vi "data_process.vi"(0 "文件（使用对话框）":path) -> (19 "SENSOR 9":dbl[](array[numeric]), 20 "SENSOR1":dbl[](array[numeric]), 21 "SENSOR 2":dbl[](array[numeric]), 22 "SENSOR 3":dbl[](array[numeric]), 23 "SENSOR 4":dbl[](array[numeric]), 24 "SENSOR 5":dbl[](array[numeric]), 25 "SENSOR 6":dbl[](array[numeric]), 26 "SENSOR 7":dbl[](array[numeric]), 27 "SENSOR 8":dbl[](array[numeric]))   [LabVIEW 2017]
panel:
  out "PWM19":dbl[](array[numeric])
  out "PWM18":dbl[](array[numeric])
  out "PWM17":dbl[](array[numeric])
  out "PWM16":dbl[](array[numeric])
  out "PWM15":dbl[](array[numeric])
  out "PWM14":dbl[](array[numeric])
  out "PWM13":dbl[](array[numeric])
  out "PWM12":dbl[](array[numeric])
  out "PWM11":dbl[](array[numeric])
  out "PWM10":dbl[](array[numeric])
  out "PWM9":dbl[](array[numeric])
  out "PWM8":dbl[](array[numeric])
  out "PWM7":dbl[](array[numeric])
  out "PWM6":dbl[](array[numeric])
  out "PWM5":dbl[](array[numeric])
  out "PWM4":dbl[](array[numeric])
  out "PWM3":dbl[](array[numeric])
  out "匹配偏移量":i32
  out "PWM2":dbl[](array[numeric])
  out "文本":string
  out "PWM1":dbl[](array[numeric])
  # "主要功能：将9行数据分别提取出来作为一个列表"
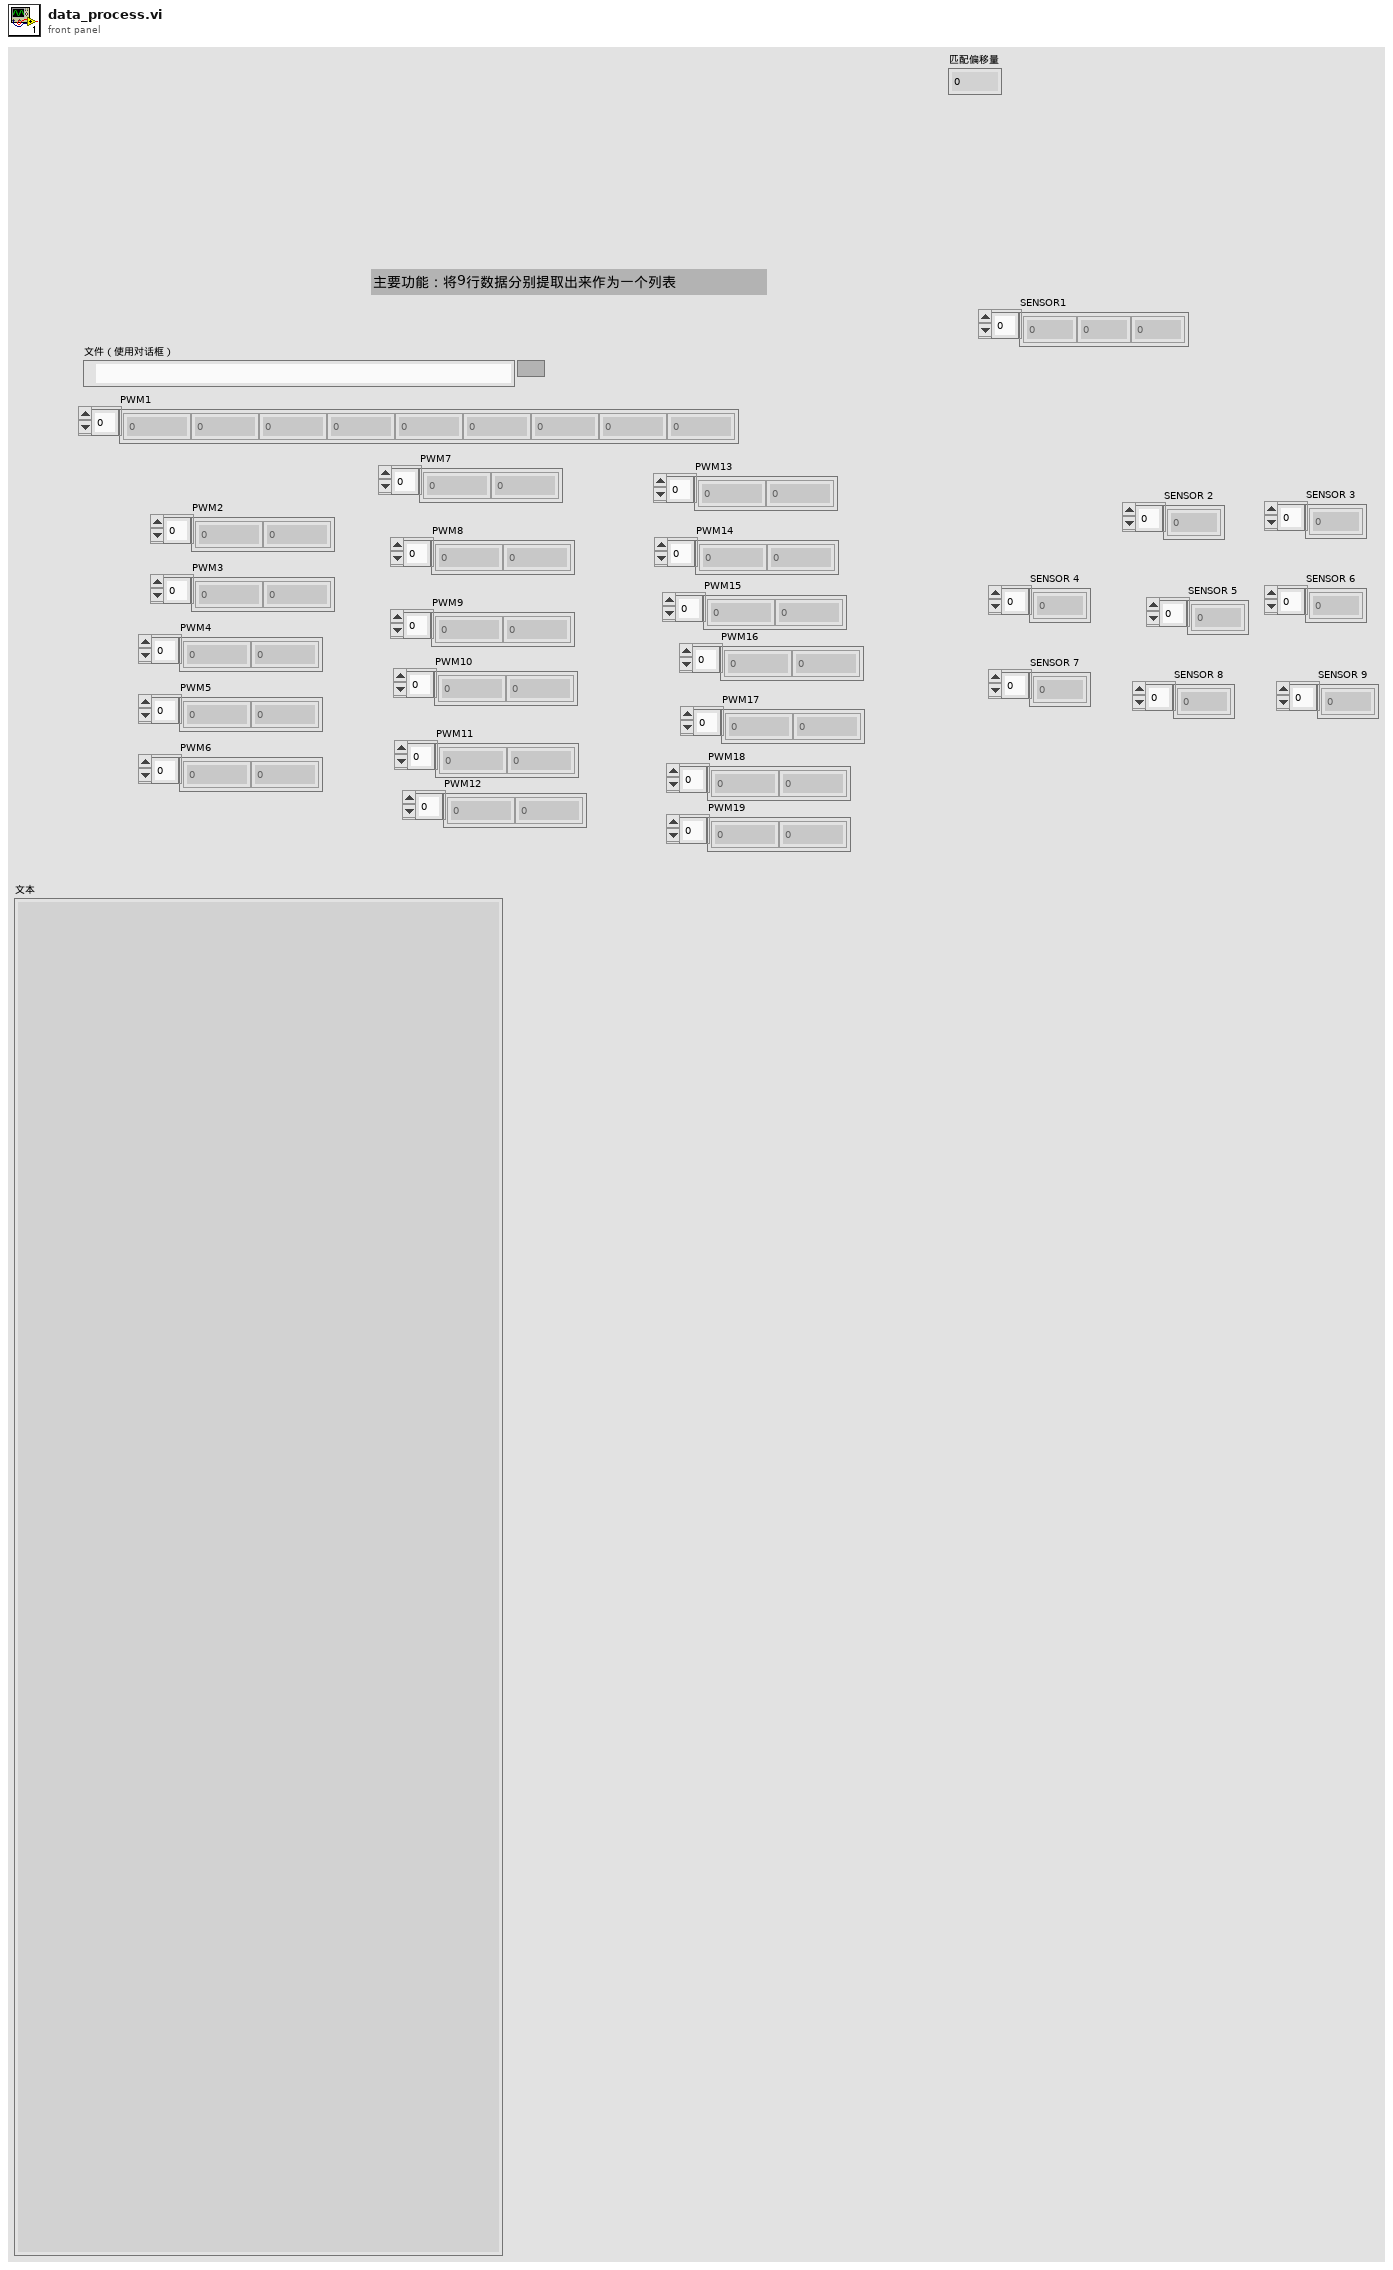
[diagram p1: front panel]
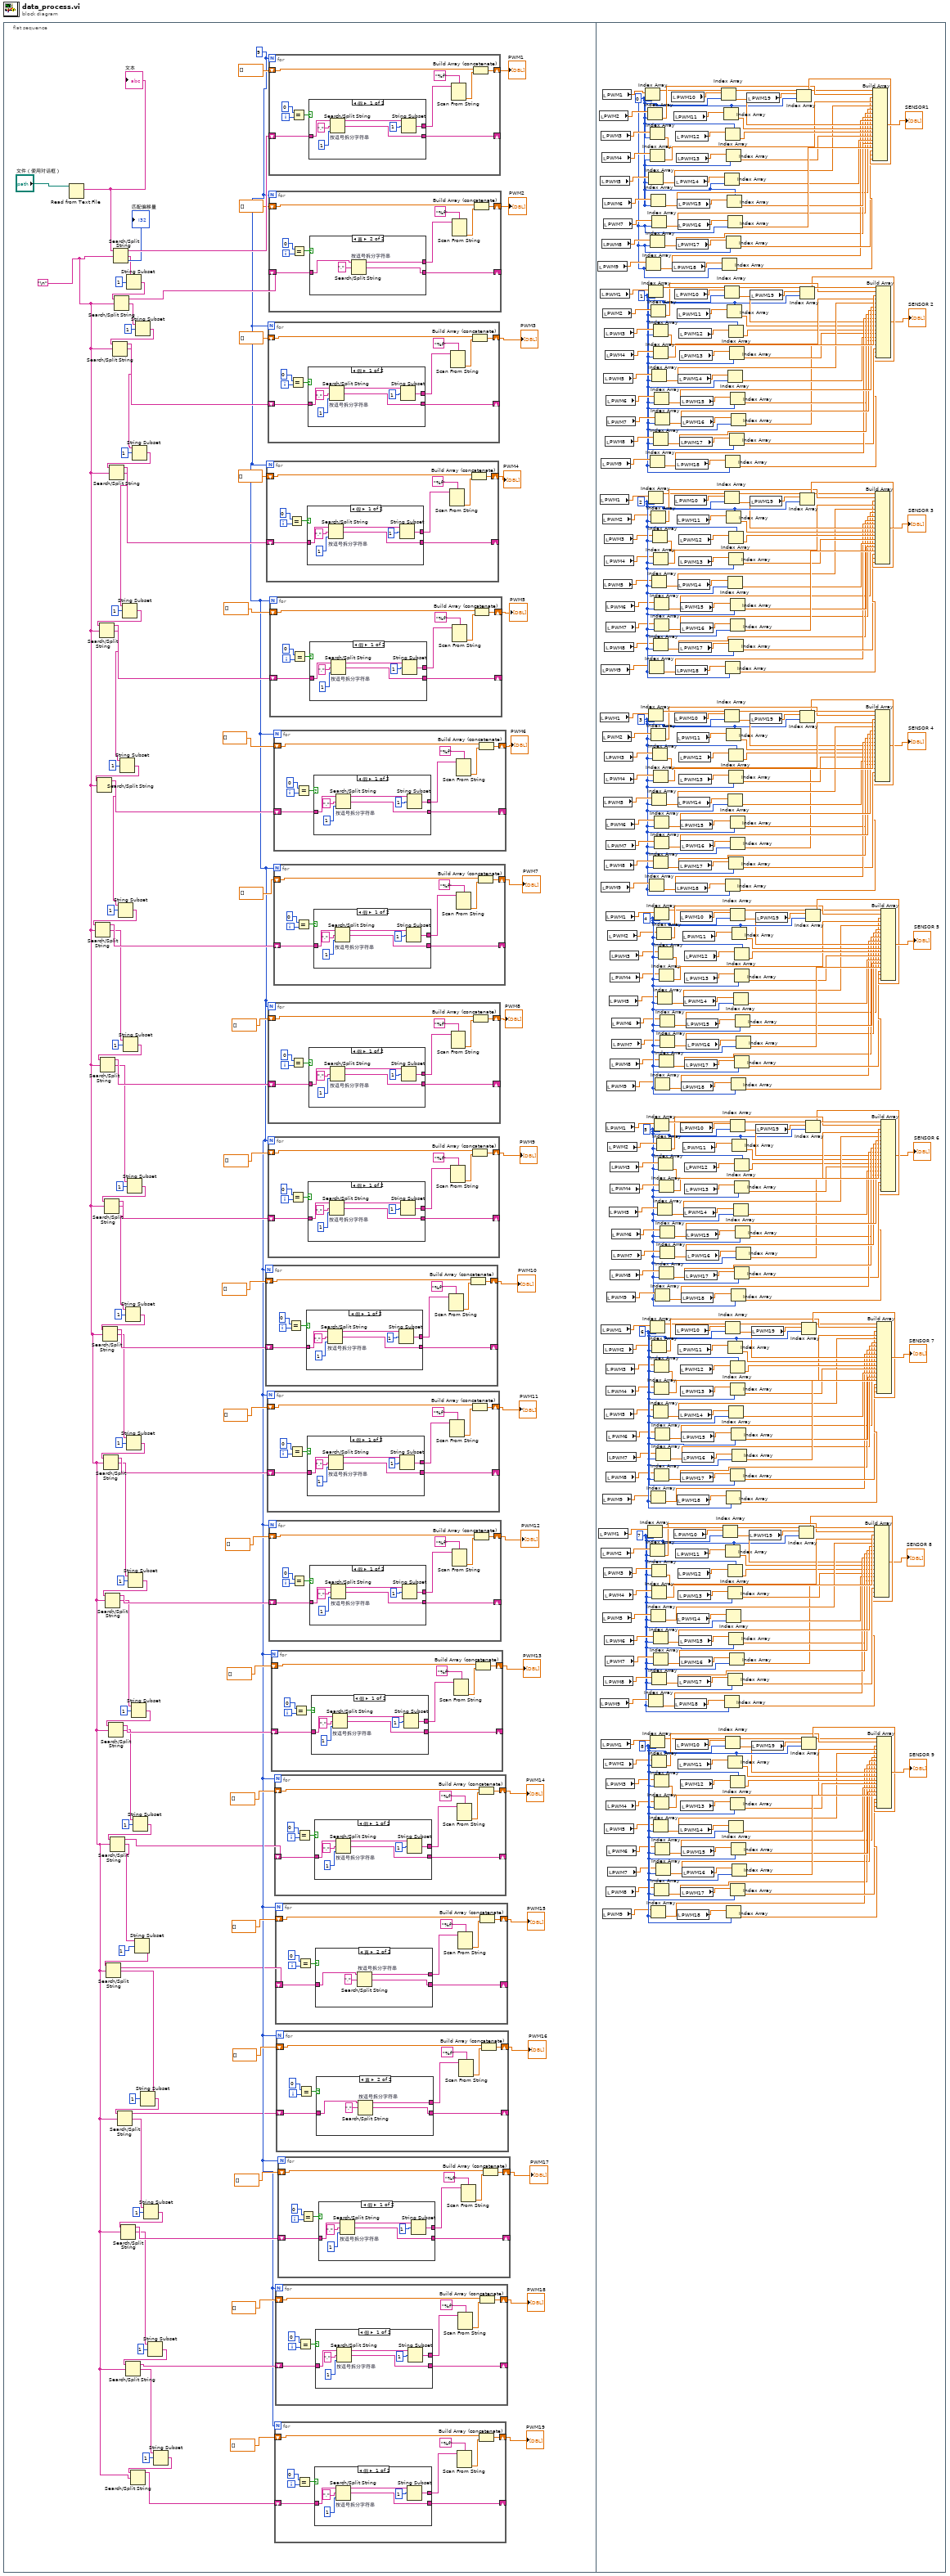
[diagram p0: block diagram]
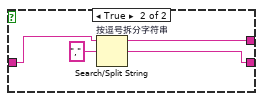
[diagram p2: hidden frame]
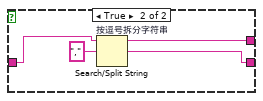
[diagram p3: hidden frame]
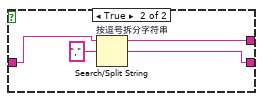
[diagram p4: hidden frame]
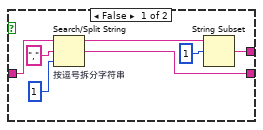
[diagram p5: hidden frame]
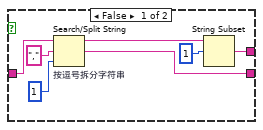
[diagram p6: hidden frame]
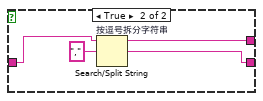
[diagram p7: hidden frame]
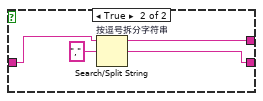
[diagram p8: hidden frame]
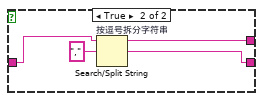
[diagram p9: hidden frame]
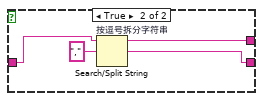
[diagram p10: hidden frame]
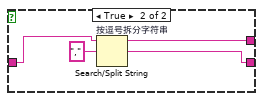
[diagram p11: hidden frame]
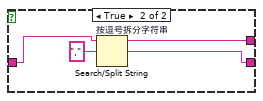
[diagram p12: hidden frame]
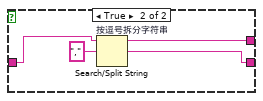
[diagram p13: hidden frame]
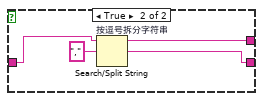
[diagram p14: hidden frame]
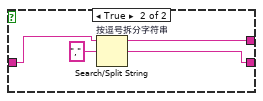
[diagram p15: hidden frame]
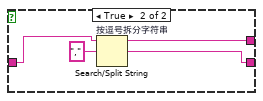
[diagram p16: hidden frame]
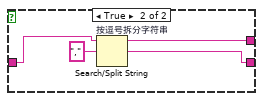
[diagram p17: hidden frame]
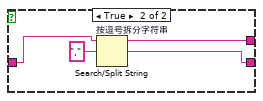
[diagram p18: hidden frame]
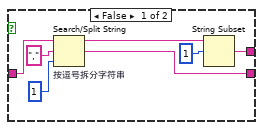
[diagram p19: hidden frame]
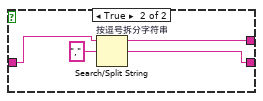
[diagram p20: hidden frame]
diagram:
  n1 = flat-sequence {
    frame #0 {
      w8 = "\n"
      w5 = 9
      n2 = Read from Text File(file (use dialog)="文件（使用对话框）") -> (text=w110:string)  [unwired: 3 in, 3 out]
      "文本" <- w110
      n3 = Search/Split String(string=w110, search string/char (-)=w8) -> (substring before match=w113:string, match + rest of string=w107:string, offset of match=→"匹配偏移量":i32)  [unwired: 1 in]
      n4 = String Subset(string=w107, offset (0)=1 ("偏移量(0)")) -> (substring=w106:string)  [unwired: 1 in]
      n5 = Search/Split String(string=w106, search string/char (-)=w8) -> (substring before match=w109:string, match + rest of string=w103:string)  [unwired: 1 in, 1 out]
      n6 = String Subset(string=w103, offset (0)=1 ("偏移量(0)")) -> (substring=w102:string)  [unwired: 1 in]
      n7 = Search/Split String(string=w102, search string/char (-)=w8) -> (substring before match=w101:string, match + rest of string=w81:string)  [unwired: 1 in, 1 out]
      n8 = String Subset(string=w81, offset (0)=1 ("偏移量(0)")) -> (substring=w85:string)  [unwired: 1 in]
      n9 = Search/Split String(string=w85, search string/char (-)=w8) -> (substring before match=w84:string, match + rest of string=w80:string)  [unwired: 1 in, 1 out]
      n10 = String Subset(string=w80, offset (0)=1 ("偏移量(0)")) -> (substring=w82:string)  [unwired: 1 in]
      n11 = Search/Split String(string=w82, search string/char (-)=w8) -> (substring before match=w79:string, match + rest of string=w76:string)  [unwired: 1 in, 1 out]
      n12 = String Subset(string=w76, offset (0)=1 ("偏移量(0)")) -> (substring=w77:string)  [unwired: 1 in]
      n13 = Search/Split String(string=w77, search string/char (-)=w8) -> (substring before match=w75:string, match + rest of string=w72:string)  [unwired: 1 in, 1 out]
      n14 = String Subset(string=w72, offset (0)=1 ("偏移量(0)")) -> (substring=w73:string)  [unwired: 1 in]
      n15 = Search/Split String(string=w73, search string/char (-)=w8) -> (substring before match=w71:string, match + rest of string=w68:string)  [unwired: 1 in, 1 out]
      n16 = String Subset(string=w68, offset (0)=1 ("偏移量(0)")) -> (substring=w69:string)  [unwired: 1 in]
      n17 = Search/Split String(string=w69, search string/char (-)=w8) -> (substring before match=w67:string, match + rest of string=w64:string)  [unwired: 1 in, 1 out]
      n18 = String Subset(string=w64, offset (0)=1 ("偏移量(0)")) -> (substring=w65:string)  [unwired: 1 in]
      n19 = Search/Split String(string=w65, search string/char (-)=w8) -> (substring before match=w63:string, match + rest of string=w41:string)  [unwired: 1 in, 1 out]
      n20 = String Subset(string=w41, offset (0)=1 ("偏移量(0)")) -> (substring=w43:string)  [unwired: 1 in]
      n21 = Search/Split String(string=w43, search string/char (-)=w8) -> (substring before match=w42:string, match + rest of string=w38:string)  [unwired: 1 in, 1 out]
      n22 = String Subset(string=w38, offset (0)=1 ("偏移量(0)")) -> (substring=w39:string)  [unwired: 1 in]
      n23 = Search/Split String(string=w39, search string/char (-)=w8) -> (substring before match=w37:string, match + rest of string=w34:string)  [unwired: 1 in, 1 out]
      n24 = String Subset(string=w34, offset (0)=1 ("偏移量(0)")) -> (substring=w35:string)  [unwired: 1 in]
      n25 = Search/Split String(string=w35, search string/char (-)=w8) -> (substring before match=w33:string, match + rest of string=w31:string)  [unwired: 1 in, 1 out]
      n26 = String Subset(string=w31, offset (0)=1 ("偏移量(0)")) -> (substring=w30:string)  [unwired: 1 in]
      n27 = Search/Split String(string=w30, search string/char (-)=w8) -> (substring before match=w27:string, match + rest of string=w26:string)  [unwired: 1 in, 1 out]
      n28 = String Subset(string=w26, offset (0)=1 ("偏移量(0)")) -> (substring=w28:string)  [unwired: 1 in]
      n29 = Search/Split String(string=w28, search string/char (-)=w8) -> (substring before match=w3:string, match + rest of string=w24:string)  [unwired: 1 in, 1 out]
      n30 = String Subset(string=w24, offset (0)=1 ("偏移量(0)")) -> (substring=w25:string)  [unwired: 1 in]
      n31 = Search/Split String(string=w25, search string/char (-)=w8) -> (substring before match=w4:string, match + rest of string=w21:string)  [unwired: 1 in, 1 out]
      n32 = String Subset(string=w21, offset (0)=1 ("偏移量(0)")) -> (substring=w22:string)  [unwired: 1 in]
      n33 = Search/Split String(string=w22, search string/char (-)=w8) -> (substring before match=w2:string, match + rest of string=w18:string)  [unwired: 1 in, 1 out]
      n34 = String Subset(string=w18, offset (0)=1 ("偏移量(0)")) -> (substring=w19:string)  [unwired: 1 in]
      n35 = Search/Split String(string=w19, search string/char (-)=w8) -> (substring before match=w17:string, match + rest of string=w14:string)  [unwired: 1 in, 1 out]
      n36 = String Subset(string=w14, offset (0)=1 ("偏移量(0)")) -> (substring=w15:string)  [unwired: 1 in]
      n37 = Search/Split String(string=w15, search string/char (-)=w8) -> (substring before match=w13:string, match + rest of string=w7:string)  [unwired: 1 in, 1 out]
      n38 = String Subset(string=w7, offset (0)=1 ("偏移量(0)")) -> (substring=w9:string)  [unwired: 1 in]
      n39 = Search/Split String(string=w9, search string/char (-)=w8) -> (substring before match=w6:string)  [unwired: 1 in, 2 out]
      n40 = for {
        N: w5 -> [_]
        shift-right: [w311] -> _
        shift-left: w42 -> [w312]
        shift-right: [w308] -> w62
        shift-left: dbl[] [] -> [w306]
        i -> [w315]
        n41 = Equal?(x=0, y=w315) -> (x = y?=w313:bool)
        n42 = case shown="假" w313 {
          tunnel: [w321 w325] -> w311
          tunnel: w312 -> [w322 w324]
          tunnel: [w316 w323] -> w309
          frame False {
            n43 = Search/Split String "按逗号拆分字符串"(string=w322, search string/char (-)="," ("搜索字符串/字符(-)"), offset (0)=1 ("偏移量(0)")) -> (substring before match=w318:string, match + rest of string=w321:string)  [unwired: 1 out]
            n44 = String Subset(string=w318, offset (0)=1 ("偏移量(0)")) -> (substring=w316:string)  [unwired: 1 in]
          }
          frame True {
            n45 = Search/Split String "按逗号拆分字符串"(string=w324, search string/char (-)="," ("搜索字符串/字符(-)")) -> (substring before match=w323:string, match + rest of string=w325:string)  [unwired: 1 in, 1 out]
          }
        }
        n46 = Scan From String(format string="%f" ("格式字符串"), input string=w309) -> (output 1=w307:dbl)  [unwired: 3 in, 3 out]
        n47 = Build Array (concatenate)(w306, w307) -> (w308:dbl[])
      }
      "PWM10" <- w62
      n48 = for {
        N: w5 -> [_]
        shift-right: [w437] -> _
        shift-left: w84 -> [w438]
        shift-right: [w434] -> w98
        shift-left: dbl[] [] -> [w432]
        i -> [w441]
        n49 = Equal?(x=0, y=w441) -> (x = y?=w439:bool)
        n50 = case shown="假" w439 {
          tunnel: [w447 w451] -> w437
          tunnel: w438 -> [w448 w450]
          tunnel: [w442 w449] -> w435
          frame False {
            n51 = Search/Split String "按逗号拆分字符串"(string=w448, search string/char (-)="," ("搜索字符串/字符(-)"), offset (0)=1 ("偏移量(0)")) -> (substring before match=w444:string, match + rest of string=w447:string)  [unwired: 1 out]
            n52 = String Subset(string=w444, offset (0)=1 ("偏移量(0)")) -> (substring=w442:string)  [unwired: 1 in]
          }
          frame True {
            n53 = Search/Split String "按逗号拆分字符串"(string=w450, search string/char (-)="," ("搜索字符串/字符(-)")) -> (substring before match=w449:string, match + rest of string=w451:string)  [unwired: 1 in, 1 out]
          }
        }
        n54 = Scan From String(format string="%f" ("格式字符串"), input string=w435) -> (output 1=w433:dbl)  [unwired: 3 in, 3 out]
        n55 = Build Array (concatenate)(w432, w433) -> (w434:dbl[])
      }
      "PWM4" <- w98
      n56 = for {
        N: w5 -> [_]
        shift-right: [w290] -> _
        shift-left: w37 -> [w291]
        shift-right: [w287] -> w60
        shift-left: dbl[] [] -> [w285]
        i -> [w294]
        n57 = Equal?(x=0, y=w294) -> (x = y?=w292:bool)
        n58 = case shown="假" w292 {
          tunnel: [w300 w304] -> w290
          tunnel: w291 -> [w301 w303]
          tunnel: [w295 w302] -> w288
          frame False {
            n59 = Search/Split String "按逗号拆分字符串"(string=w301, search string/char (-)="," ("搜索字符串/字符(-)"), offset (0)=1 ("偏移量(0)")) -> (substring before match=w297:string, match + rest of string=w300:string)  [unwired: 1 out]
            n60 = String Subset(string=w297, offset (0)=1 ("偏移量(0)")) -> (substring=w295:string)  [unwired: 1 in]
          }
          frame True {
            n61 = Search/Split String "按逗号拆分字符串"(string=w303, search string/char (-)="," ("搜索字符串/字符(-)")) -> (substring before match=w302:string, match + rest of string=w304:string)  [unwired: 1 in, 1 out]
          }
        }
        n62 = Scan From String(format string="%f" ("格式字符串"), input string=w288) -> (output 1=w286:dbl)  [unwired: 3 in, 3 out]
        n63 = Build Array (concatenate)(w285, w286) -> (w287:dbl[])
      }
      "PWM11" <- w60
      n64 = for {
        N: w5 -> [_]
        shift-right: [w458] -> _
        shift-left: w101 -> [w459]
        shift-right: [w455] -> w99
        shift-left: dbl[] [] -> [w453]
        i -> [w462]
        n65 = Equal?(x=0, y=w462) -> (x = y?=w460:bool)
        n66 = case shown="假" w460 {
          tunnel: [w468 w472] -> w458
          tunnel: w459 -> [w469 w471]
          tunnel: [w463 w470] -> w456
          frame False {
            n67 = Search/Split String "按逗号拆分字符串"(string=w469, search string/char (-)="," ("搜索字符串/字符(-)"), offset (0)=1 ("偏移量(0)")) -> (substring before match=w465:string, match + rest of string=w468:string)  [unwired: 1 out]
            n68 = String Subset(string=w465, offset (0)=1 ("偏移量(0)")) -> (substring=w463:string)  [unwired: 1 in]
          }
          frame True {
            n69 = Search/Split String "按逗号拆分字符串"(string=w471, search string/char (-)="," ("搜索字符串/字符(-)")) -> (substring before match=w470:string, match + rest of string=w472:string)  [unwired: 1 in, 1 out]
          }
        }
        n70 = Scan From String(format string="%f" ("格式字符串"), input string=w456) -> (output 1=w454:dbl)  [unwired: 3 in, 3 out]
        n71 = Build Array (concatenate)(w453, w454) -> (w455:dbl[])
      }
      "PWM3" <- w99
      n72 = for {
        N: w5 -> [_]
        shift-right: [w332] -> _
        shift-left: w63 -> [w333]
        shift-right: [w329] -> w93
        shift-left: dbl[] [] -> [w327]
        i -> [w336]
        n73 = Equal?(x=0, y=w336) -> (x = y?=w334:bool)
        n74 = case shown="假" w334 {
          tunnel: [w342 w346] -> w332
          tunnel: w333 -> [w343 w345]
          tunnel: [w337 w344] -> w330
          frame False {
            n75 = Search/Split String "按逗号拆分字符串"(string=w343, search string/char (-)="," ("搜索字符串/字符(-)"), offset (0)=1 ("偏移量(0)")) -> (substring before match=w339:string, match + rest of string=w342:string)  [unwired: 1 out]
            n76 = String Subset(string=w339, offset (0)=1 ("偏移量(0)")) -> (substring=w337:string)  [unwired: 1 in]
          }
          frame True {
            n77 = Search/Split String "按逗号拆分字符串"(string=w345, search string/char (-)="," ("搜索字符串/字符(-)")) -> (substring before match=w344:string, match + rest of string=w346:string)  [unwired: 1 in, 1 out]
          }
        }
        n78 = Scan From String(format string="%f" ("格式字符串"), input string=w330) -> (output 1=w328:dbl)  [unwired: 3 in, 3 out]
        n79 = Build Array (concatenate)(w327, w328) -> (w329:dbl[])
      }
      "PWM9" <- w93
      n80 = for {
        N: w5 -> [_]
        shift-right: [w353] -> _
        shift-left: w67 -> [w354]
        shift-right: [w350] -> w94
        shift-left: dbl[] [] -> [w348]
        i -> [w357]
        n81 = Equal?(x=0, y=w357) -> (x = y?=w355:bool)
        n82 = case shown="假" w355 {
          tunnel: [w363 w367] -> w353
          tunnel: w354 -> [w364 w366]
          tunnel: [w358 w365] -> w351
          frame False {
            n83 = Search/Split String "按逗号拆分字符串"(string=w364, search string/char (-)="," ("搜索字符串/字符(-)"), offset (0)=1 ("偏移量(0)")) -> (substring before match=w360:string, match + rest of string=w363:string)  [unwired: 1 out]
            n84 = String Subset(string=w360, offset (0)=1 ("偏移量(0)")) -> (substring=w358:string)  [unwired: 1 in]
          }
          frame True {
            n85 = Search/Split String "按逗号拆分字符串"(string=w366, search string/char (-)="," ("搜索字符串/字符(-)")) -> (substring before match=w365:string, match + rest of string=w367:string)  [unwired: 1 in, 1 out]
          }
        }
        n86 = Scan From String(format string="%f" ("格式字符串"), input string=w351) -> (output 1=w349:dbl)  [unwired: 3 in, 3 out]
        n87 = Build Array (concatenate)(w348, w349) -> (w350:dbl[])
      }
      "PWM8" <- w94
      n88 = for {
        N: w5 -> [_]
        shift-right: [w500] -> _
        shift-left: w113 -> [w501]
        shift-right: [w497] -> w114
        shift-left: dbl[] [] -> [w495]
        i -> [w504]
        n89 = Equal?(x=0, y=w504) -> (x = y?=w502:bool)
        n90 = case shown="假" w502 {
          tunnel: [w510 w514] -> w500
          tunnel: w501 -> [w511 w513]
          tunnel: [w505 w512] -> w498
          frame False {
            n91 = Search/Split String "按逗号拆分字符串"(string=w511, search string/char (-)="," ("搜索字符串/字符(-)"), offset (0)=1 ("偏移量(0)")) -> (substring before match=w507:string, match + rest of string=w510:string)  [unwired: 1 out]
            n92 = String Subset(string=w507, offset (0)=1 ("偏移量(0)")) -> (substring=w505:string)  [unwired: 1 in]
          }
          frame True {
            n93 = Search/Split String "按逗号拆分字符串"(string=w513, search string/char (-)="," ("搜索字符串/字符(-)")) -> (substring before match=w512:string, match + rest of string=w514:string)  [unwired: 1 in, 1 out]
          }
        }
        n94 = Scan From String(format string="%f" ("格式字符串"), input string=w498) -> (output 1=w496:dbl)  [unwired: 3 in, 3 out]
        n95 = Build Array (concatenate)(w495, w496) -> (w497:dbl[])
      }
      "PWM1" <- w114
      n96 = for {
        N: w5 -> [_]
        shift-right: [w479] -> _
        shift-left: w109 -> [w480]
        shift-right: [w476] -> w111
        shift-left: dbl[] [] -> [w474]
        i -> [w483]
        n97 = Equal?(x=0, y=w483) -> (x = y?=w481:bool)
        n98 = case shown="真" w481 {
          tunnel: [w489 w493] -> w479
          tunnel: w480 -> [w490 w492]
          tunnel: [w484 w491] -> w477
          frame False {
            n99 = Search/Split String "按逗号拆分字符串"(string=w490, search string/char (-)="," ("搜索字符串/字符(-)"), offset (0)=1 ("偏移量(0)")) -> (substring before match=w486:string, match + rest of string=w489:string)  [unwired: 1 out]
            n100 = String Subset(string=w486, offset (0)=1 ("偏移量(0)")) -> (substring=w484:string)  [unwired: 1 in]
          }
          frame True {
            n101 = Search/Split String "按逗号拆分字符串"(string=w492, search string/char (-)="," ("搜索字符串/字符(-)")) -> (substring before match=w491:string, match + rest of string=w493:string)  [unwired: 1 in, 1 out]
          }
        }
        n102 = Scan From String(format string="%f" ("格式字符串"), input string=w477) -> (output 1=w475:dbl)  [unwired: 3 in, 3 out]
        n103 = Build Array (concatenate)(w474, w475) -> (w476:dbl[])
      }
      "PWM2" <- w111
      n104 = for {
        N: w5 -> [_]
        shift-right: [w269] -> _
        shift-left: w33 -> [w270]
        shift-right: [w266] -> w58
        shift-left: dbl[] [] -> [w264]
        i -> [w273]
        n105 = Equal?(x=0, y=w273) -> (x = y?=w271:bool)
        n106 = case shown="假" w271 {
          tunnel: [w279 w283] -> w269
          tunnel: w270 -> [w280 w282]
          tunnel: [w274 w281] -> w267
          frame False {
            n107 = Search/Split String "按逗号拆分字符串"(string=w280, search string/char (-)="," ("搜索字符串/字符(-)"), offset (0)=1 ("偏移量(0)")) -> (substring before match=w276:string, match + rest of string=w279:string)  [unwired: 1 out]
            n108 = String Subset(string=w276, offset (0)=1 ("偏移量(0)")) -> (substring=w274:string)  [unwired: 1 in]
          }
          frame True {
            n109 = Search/Split String "按逗号拆分字符串"(string=w282, search string/char (-)="," ("搜索字符串/字符(-)")) -> (substring before match=w281:string, match + rest of string=w283:string)  [unwired: 1 in, 1 out]
          }
        }
        n110 = Scan From String(format string="%f" ("格式字符串"), input string=w267) -> (output 1=w265:dbl)  [unwired: 3 in, 3 out]
        n111 = Build Array (concatenate)(w264, w265) -> (w266:dbl[])
      }
      "PWM12" <- w58
      n112 = for {
        N: w5 -> [_]
        shift-right: [w416] -> _
        shift-left: w79 -> [w417]
        shift-right: [w413] -> w97
        shift-left: dbl[] [] -> [w411]
        i -> [w420]
        n113 = Equal?(x=0, y=w420) -> (x = y?=w418:bool)
        n114 = case shown="假" w418 {
          tunnel: [w426 w430] -> w416
          tunnel: w417 -> [w427 w429]
          tunnel: [w421 w428] -> w414
          frame False {
            n115 = Search/Split String "按逗号拆分字符串"(string=w427, search string/char (-)="," ("搜索字符串/字符(-)"), offset (0)=1 ("偏移量(0)")) -> (substring before match=w423:string, match + rest of string=w426:string)  [unwired: 1 out]
            n116 = String Subset(string=w423, offset (0)=1 ("偏移量(0)")) -> (substring=w421:string)  [unwired: 1 in]
          }
          frame True {
            n117 = Search/Split String "按逗号拆分字符串"(string=w429, search string/char (-)="," ("搜索字符串/字符(-)")) -> (substring before match=w428:string, match + rest of string=w430:string)  [unwired: 1 in, 1 out]
          }
        }
        n118 = Scan From String(format string="%f" ("格式字符串"), input string=w414) -> (output 1=w412:dbl)  [unwired: 3 in, 3 out]
        n119 = Build Array (concatenate)(w411, w412) -> (w413:dbl[])
      }
      "PWM5" <- w97
      n120 = for {
        N: w5 -> [_]
        shift-right: [w248] -> _
        shift-left: w27 -> [w249]
        shift-right: [w245] -> w56
        shift-left: dbl[] [] -> [w243]
        i -> [w252]
        n121 = Equal?(x=0, y=w252) -> (x = y?=w250:bool)
        n122 = case shown="假" w250 {
          tunnel: [w258 w262] -> w248
          tunnel: w249 -> [w259 w261]
          tunnel: [w253 w260] -> w246
          frame False {
            n123 = Search/Split String "按逗号拆分字符串"(string=w259, search string/char (-)="," ("搜索字符串/字符(-)"), offset (0)=1 ("偏移量(0)")) -> (substring before match=w255:string, match + rest of string=w258:string)  [unwired: 1 out]
            n124 = String Subset(string=w255, offset (0)=1 ("偏移量(0)")) -> (substring=w253:string)  [unwired: 1 in]
          }
          frame True {
            n125 = Search/Split String "按逗号拆分字符串"(string=w261, search string/char (-)="," ("搜索字符串/字符(-)")) -> (substring before match=w260:string, match + rest of string=w262:string)  [unwired: 1 in, 1 out]
          }
        }
        n126 = Scan From String(format string="%f" ("格式字符串"), input string=w246) -> (output 1=w244:dbl)  [unwired: 3 in, 3 out]
        n127 = Build Array (concatenate)(w243, w244) -> (w245:dbl[])
      }
      "PWM13" <- w56
      n128 = for {
        N: w5 -> [_]
        shift-right: [w374] -> _
        shift-left: w71 -> [w375]
        shift-right: [w371] -> w95
        shift-left: dbl[] [] -> [w369]
        i -> [w378]
        n129 = Equal?(x=0, y=w378) -> (x = y?=w376:bool)
        n130 = case shown="假" w376 {
          tunnel: [w384 w388] -> w374
          tunnel: w375 -> [w385 w387]
          tunnel: [w379 w386] -> w372
          frame False {
            n131 = Search/Split String "按逗号拆分字符串"(string=w385, search string/char (-)="," ("搜索字符串/字符(-)"), offset (0)=1 ("偏移量(0)")) -> (substring before match=w381:string, match + rest of string=w384:string)  [unwired: 1 out]
            n132 = String Subset(string=w381, offset (0)=1 ("偏移量(0)")) -> (substring=w379:string)  [unwired: 1 in]
          }
          frame True {
            n133 = Search/Split String "按逗号拆分字符串"(string=w387, search string/char (-)="," ("搜索字符串/字符(-)")) -> (substring before match=w386:string, match + rest of string=w388:string)  [unwired: 1 in, 1 out]
          }
        }
        n134 = Scan From String(format string="%f" ("格式字符串"), input string=w372) -> (output 1=w370:dbl)  [unwired: 3 in, 3 out]
        n135 = Build Array (concatenate)(w369, w370) -> (w371:dbl[])
      }
      "PWM7" <- w95
      n136 = for {
        N: w5 -> [_]
        shift-right: [w395] -> _
        shift-left: w75 -> [w396]
        shift-right: [w392] -> w96
        shift-left: dbl[] [] -> [w390]
        i -> [w399]
        n137 = Equal?(x=0, y=w399) -> (x = y?=w397:bool)
        n138 = case shown="假" w397 {
          tunnel: [w405 w409] -> w395
          tunnel: w396 -> [w406 w408]
          tunnel: [w400 w407] -> w393
          frame False {
            n139 = Search/Split String "按逗号拆分字符串"(string=w406, search string/char (-)="," ("搜索字符串/字符(-)"), offset (0)=1 ("偏移量(0)")) -> (substring before match=w402:string, match + rest of string=w405:string)  [unwired: 1 out]
            n140 = String Subset(string=w402, offset (0)=1 ("偏移量(0)")) -> (substring=w400:string)  [unwired: 1 in]
          }
          frame True {
            n141 = Search/Split String "按逗号拆分字符串"(string=w408, search string/char (-)="," ("搜索字符串/字符(-)")) -> (substring before match=w407:string, match + rest of string=w409:string)  [unwired: 1 in, 1 out]
          }
        }
        n142 = Scan From String(format string="%f" ("格式字符串"), input string=w393) -> (output 1=w391:dbl)  [unwired: 3 in, 3 out]
        n143 = Build Array (concatenate)(w390, w391) -> (w392:dbl[])
      }
      "PWM6" <- w96
      n144 = for {
        N: w5 -> [_]
        shift-right: [w227] -> _
        shift-left: w3 -> [w228]
        shift-right: [w224] -> w54
        shift-left: dbl[] [] -> [w222]
        i -> [w231]
        n145 = Equal?(x=0, y=w231) -> (x = y?=w229:bool)
        n146 = case shown="假" w229 {
          tunnel: [w237 w241] -> w227
          tunnel: w228 -> [w238 w240]
          tunnel: [w232 w239] -> w225
          frame False {
            n147 = Search/Split String "按逗号拆分字符串"(string=w238, search string/char (-)="," ("搜索字符串/字符(-)"), offset (0)=1 ("偏移量(0)")) -> (substring before match=w234:string, match + rest of string=w237:string)  [unwired: 1 out]
            n148 = String Subset(string=w234, offset (0)=1 ("偏移量(0)")) -> (substring=w232:string)  [unwired: 1 in]
          }
          frame True {
            n149 = Search/Split String "按逗号拆分字符串"(string=w240, search string/char (-)="," ("搜索字符串/字符(-)")) -> (substring before match=w239:string, match + rest of string=w241:string)  [unwired: 1 in, 1 out]
          }
        }
        n150 = Scan From String(format string="%f" ("格式字符串"), input string=w225) -> (output 1=w223:dbl)  [unwired: 3 in, 3 out]
        n151 = Build Array (concatenate)(w222, w223) -> (w224:dbl[])
      }
      "PWM14" <- w54
      n152 = for {
        N: w5 -> [_]
        shift-right: [w122] -> _
        shift-left: w6 -> [w123]
        shift-right: [w119] -> w12
        shift-left: dbl[] [] -> [w117]
        i -> [w126]
        n153 = Equal?(x=0, y=w126) -> (x = y?=w124:bool)
        n154 = case shown="假" w124 {
          tunnel: [w132 w136] -> w122
          tunnel: w123 -> [w133 w135]
          tunnel: [w127 w134] -> w120
          frame False {
            n155 = Search/Split String "按逗号拆分字符串"(string=w133, search string/char (-)="," ("搜索字符串/字符(-)"), offset (0)=1 ("偏移量(0)")) -> (substring before match=w129:string, match + rest of string=w132:string)  [unwired: 1 out]
            n156 = String Subset(string=w129, offset (0)=1 ("偏移量(0)")) -> (substring=w127:string)  [unwired: 1 in]
          }
          frame True {
            n157 = Search/Split String "按逗号拆分字符串"(string=w135, search string/char (-)="," ("搜索字符串/字符(-)")) -> (substring before match=w134:string, match + rest of string=w136:string)  [unwired: 1 in, 1 out]
          }
        }
        n158 = Scan From String(format string="%f" ("格式字符串"), input string=w120) -> (output 1=w118:dbl)  [unwired: 3 in, 3 out]
        n159 = Build Array (concatenate)(w117, w118) -> (w119:dbl[])
      }
      "PWM19" <- w12
      n160 = for {
        N: w5 -> [_]
        shift-right: [w206] -> _
        shift-left: w4 -> [w207]
        shift-right: [w203] -> w52
        shift-left: dbl[] [] -> [w201]
        i -> [w210]
        n161 = Equal?(x=0, y=w210) -> (x = y?=w208:bool)
        n162 = case shown="真" w208 {
          tunnel: [w216 w220] -> w206
          tunnel: w207 -> [w217 w219]
          tunnel: [w211 w218] -> w204
          frame False {
            n163 = Search/Split String "按逗号拆分字符串"(string=w217, search string/char (-)="," ("搜索字符串/字符(-)"), offset (0)=1 ("偏移量(0)")) -> (substring before match=w213:string, match + rest of string=w216:string)  [unwired: 1 out]
            n164 = String Subset(string=w213, offset (0)=1 ("偏移量(0)")) -> (substring=w211:string)  [unwired: 1 in]
          }
          frame True {
            n165 = Search/Split String "按逗号拆分字符串"(string=w219, search string/char (-)="," ("搜索字符串/字符(-)")) -> (substring before match=w218:string, match + rest of string=w220:string)  [unwired: 1 in, 1 out]
          }
        }
        n166 = Scan From String(format string="%f" ("格式字符串"), input string=w204) -> (output 1=w202:dbl)  [unwired: 3 in, 3 out]
        n167 = Build Array (concatenate)(w201, w202) -> (w203:dbl[])
      }
      "PWM15" <- w52
      n168 = for {
        N: w5 -> [_]
        shift-right: [w143] -> _
        shift-left: w13 -> [w144]
        shift-right: [w140] -> w46
        shift-left: dbl[] [] -> [w138]
        i -> [w147]
        n169 = Equal?(x=0, y=w147) -> (x = y?=w145:bool)
        n170 = case shown="假" w145 {
          tunnel: [w153 w157] -> w143
          tunnel: w144 -> [w154 w156]
          tunnel: [w148 w155] -> w141
          frame False {
            n171 = Search/Split String "按逗号拆分字符串"(string=w154, search string/char (-)="," ("搜索字符串/字符(-)"), offset (0)=1 ("偏移量(0)")) -> (substring before match=w150:string, match + rest of string=w153:string)  [unwired: 1 out]
            n172 = String Subset(string=w150, offset (0)=1 ("偏移量(0)")) -> (substring=w148:string)  [unwired: 1 in]
          }
          frame True {
            n173 = Search/Split String "按逗号拆分字符串"(string=w156, search string/char (-)="," ("搜索字符串/字符(-)")) -> (substring before match=w155:string, match + rest of string=w157:string)  [unwired: 1 in, 1 out]
          }
        }
        n174 = Scan From String(format string="%f" ("格式字符串"), input string=w141) -> (output 1=w139:dbl)  [unwired: 3 in, 3 out]
        n175 = Build Array (concatenate)(w138, w139) -> (w140:dbl[])
      }
      "PWM18" <- w46
      n176 = for {
        N: w5 -> [_]
        shift-right: [w185] -> _
        shift-left: w2 -> [w186]
        shift-right: [w182] -> w50
        shift-left: dbl[] [] -> [w180]
        i -> [w189]
        n177 = Equal?(x=0, y=w189) -> (x = y?=w187:bool)
        n178 = case shown="真" w187 {
          tunnel: [w195 w199] -> w185
          tunnel: w186 -> [w196 w198]
          tunnel: [w190 w197] -> w183
          frame False {
            n179 = Search/Split String "按逗号拆分字符串"(string=w196, search string/char (-)="," ("搜索字符串/字符(-)"), offset (0)=1 ("偏移量(0)")) -> (substring before match=w192:string, match + rest of string=w195:string)  [unwired: 1 out]
            n180 = String Subset(string=w192, offset (0)=1 ("偏移量(0)")) -> (substring=w190:string)  [unwired: 1 in]
          }
          frame True {
            n181 = Search/Split String "按逗号拆分字符串"(string=w198, search string/char (-)="," ("搜索字符串/字符(-)")) -> (substring before match=w197:string, match + rest of string=w199:string)  [unwired: 1 in, 1 out]
          }
        }
        n182 = Scan From String(format string="%f" ("格式字符串"), input string=w183) -> (output 1=w181:dbl)  [unwired: 3 in, 3 out]
        n183 = Build Array (concatenate)(w180, w181) -> (w182:dbl[])
      }
      "PWM16" <- w50
      n184 = for {
        N: w5 -> [_]
        shift-right: [w164] -> _
        shift-left: w17 -> [w165]
        shift-right: [w161] -> w48
        shift-left: dbl[] [] -> [w159]
        i -> [w168]
        n185 = Equal?(x=0, y=w168) -> (x = y?=w166:bool)
        n186 = case shown="假" w166 {
          tunnel: [w174 w178] -> w164
          tunnel: w165 -> [w175 w177]
          tunnel: [w169 w176] -> w162
          frame False {
            n187 = Search/Split String "按逗号拆分字符串"(string=w175, search string/char (-)="," ("搜索字符串/字符(-)"), offset (0)=1 ("偏移量(0)")) -> (substring before match=w171:string, match + rest of string=w174:string)  [unwired: 1 out]
            n188 = String Subset(string=w171, offset (0)=1 ("偏移量(0)")) -> (substring=w169:string)  [unwired: 1 in]
          }
          frame True {
            n189 = Search/Split String "按逗号拆分字符串"(string=w177, search string/char (-)="," ("搜索字符串/字符(-)")) -> (substring before match=w176:string, match + rest of string=w178:string)  [unwired: 1 in, 1 out]
          }
        }
        n190 = Scan From String(format string="%f" ("格式字符串"), input string=w162) -> (output 1=w160:dbl)  [unwired: 3 in, 3 out]
        n191 = Build Array (concatenate)(w159, w160) -> (w161:dbl[])
      }
      "PWM17" <- w48
    }
    frame #1 {
      w555 = 8 ("索引")
      w556 = 7 ("索引")
      w635 = 6 ("索引")
      w636 = 5 ("索引")
      w715 = 4 ("索引")
      w716 = 3 ("索引")
      w795 = 2 ("索引")
      w797 = 1 ("索引")
      w796 = 0 ("索引")
      n192 = local read "PWM9"() -> (w806:dbl[])
      n193 = local read "PWM1"() -> (w595:dbl[])
      n194 = local read "PWM2"() -> (w799:dbl[])
      n195 = local read "PWM1"() -> (w756:dbl[])
      n196 = local read "PWM1"() -> (w755:dbl[])
      n197 = local read "PWM9"() -> (w586:dbl[])
      n198 = local read "PWM5"() -> (w802:dbl[])
      n199 = local read "PWM1"() -> (w874:dbl[])
      n200 = local read "PWM9"() -> (w765:dbl[])
      n201 = local read "PWM9"() -> (w746:dbl[])
      n202 = local read "PWM3"() -> (w800:dbl[])
      n203 = local read "PWM9"() -> (w865:dbl[])
      n204 = local read "PWM1"() -> (w596:dbl[])
      n205 = local read "PWM2"() -> (w593:dbl[])
      n206 = local read "PWM1"() -> (w516:dbl[])
      n207 = local read "PWM4"() -> (w801:dbl[])
      n208 = local read "PWM8"() -> (w805:dbl[])
      n209 = local read "PWM1"() -> (w875:dbl[])
      n210 = local read "PWM2"() -> (w758:dbl[])
      n211 = local read "PWM2"() -> (w753:dbl[])
      n212 = local read "PWM9"() -> (w605:dbl[])
      n213 = local read "PWM5"() -> (w590:dbl[])
      n214 = local read "PWM9"() -> (w525:dbl[])
      n215 = local read "PWM6"() -> (w803:dbl[])
      n216 = local read "PWM2"() -> (w872:dbl[])
      n217 = local read "PWM7"() -> (w804:dbl[])
      n218 = local read "PWM5"() -> (w761:dbl[])
      n219 = local read "PWM5"() -> (w750:dbl[])
      n220 = local read "PWM3"() -> (w592:dbl[])
      n221 = local read "PWM5"() -> (w869:dbl[])
      n222 = local read "PWM2"() -> (w598:dbl[])
      n223 = local read "PWM4"() -> (w591:dbl[])
      n224 = local read "PWM8"() -> (w587:dbl[])
      n225 = local read "PWM2"() -> (w518:dbl[])
      n226 = local read "PWM3"() -> (w759:dbl[])
      n227 = local read "PWM3"() -> (w752:dbl[])
      n228 = local read "PWM3"() -> (w871:dbl[])
      n229 = local read "PWM4"() -> (w760:dbl[])
      n230 = local read "PWM8"() -> (w764:dbl[])
      n231 = local read "PWM4"() -> (w751:dbl[])
      n232 = local read "PWM8"() -> (w747:dbl[])
      n233 = local read "PWM5"() -> (w601:dbl[])
      n234 = local read "PWM6"() -> (w589:dbl[])
      n235 = local read "PWM5"() -> (w521:dbl[])
      n236 = local read "PWM4"() -> (w870:dbl[])
      n237 = local read "PWM8"() -> (w866:dbl[])
      n238 = local read "PWM7"() -> (w588:dbl[])
      n239 = local read "PWM6"() -> (w762:dbl[])
      n240 = local read "PWM6"() -> (w749:dbl[])
      n241 = local read "PWM1"() -> (w676:dbl[])
      n242 = local read "PWM1"() -> (w675:dbl[])
      n243 = local read "PWM3"() -> (w599:dbl[])
      n244 = local read "PWM3"() -> (w519:dbl[])
      n245 = local read "PWM6"() -> (w868:dbl[])
      n246 = local read "PWM7"() -> (w763:dbl[])
      n247 = local read "PWM7"() -> (w748:dbl[])
      n248 = local read "PWM4"() -> (w600:dbl[])
      n249 = local read "PWM8"() -> (w604:dbl[])
      n250 = local read "PWM4"() -> (w520:dbl[])
      n251 = local read "PWM8"() -> (w524:dbl[])
      n252 = local read "PWM7"() -> (w867:dbl[])
      n253 = local read "PWM9"() -> (w685:dbl[])
      n254 = local read "PWM9"() -> (w666:dbl[])
      n255 = local read "PWM6"() -> (w602:dbl[])
      n256 = local read "PWM6"() -> (w522:dbl[])
      n257 = local read "PWM7"() -> (w603:dbl[])
      n258 = local read "PWM7"() -> (w523:dbl[])
      n259 = local read "PWM2"() -> (w678:dbl[])
      n260 = local read "PWM2"() -> (w673:dbl[])
      n261 = local read "PWM5"() -> (w681:dbl[])
      n262 = local read "PWM5"() -> (w670:dbl[])
      n263 = local read "PWM3"() -> (w679:dbl[])
      n264 = local read "PWM3"() -> (w672:dbl[])
      n265 = local read "PWM4"() -> (w680:dbl[])
      n266 = local read "PWM8"() -> (w684:dbl[])
      n267 = local read "PWM4"() -> (w671:dbl[])
      n268 = local read "PWM8"() -> (w667:dbl[])
      n269 = local read "PWM6"() -> (w682:dbl[])
      n270 = local read "PWM6"() -> (w669:dbl[])
      n271 = local read "PWM7"() -> (w683:dbl[])
      n272 = local read "PWM7"() -> (w668:dbl[])
      n273 = Index Array(array=w875, index=w796) -> (element=w798:dbl)
      n274 = Index Array(array=w806, index=w796) -> (element=w824:dbl)
      n275 = Index Array(array=w595, index=w556) -> (element=w594:dbl)
      n276 = Index Array(array=w799, index=w796) -> (element=w817:dbl)
      n277 = Index Array(array=w756, index=w795) -> (element=w757:dbl)
      n278 = Index Array(array=w755, index=w716) -> (element=w754:dbl)
      n279 = Index Array(array=w586, index=w556) -> (element=w568:dbl)
      n280 = Index Array(array=w802, index=w796) -> (element=w820:dbl)
      n281 = Index Array(array=w874, index=w797) -> (element=w873:dbl)
      n282 = Index Array(array=w765, index=w795) -> (element=w783:dbl)
      n283 = Index Array(array=w746, index=w716) -> (element=w728:dbl)
      n284 = Index Array(array=w800, index=w796) -> (element=w818:dbl)
      n285 = Index Array(array=w865, index=w797) -> (element=w847:dbl)
      n286 = Index Array(array=w596, index=w635) -> (element=w597:dbl)
      n287 = Index Array(array=w593, index=w556) -> (element=w575:dbl)
      n288 = Index Array(array=w516, index=w555) -> (element=w517:dbl)
      n289 = Index Array(array=w801, index=w796) -> (element=w819:dbl)
      n290 = Index Array(array=w805, index=w796) -> (element=w823:dbl)
      n291 = Index Array(array=w758, index=w795) -> (element=w776:dbl)
      n292 = Index Array(array=w753, index=w716) -> (element=w735:dbl)
      n293 = Index Array(array=w605, index=w635) -> (element=w623:dbl)
      n294 = Index Array(array=w590, index=w556) -> (element=w572:dbl)
      n295 = Index Array(array=w525, index=w555) -> (element=w543:dbl)
      n296 = Index Array(array=w803, index=w796) -> (element=w821:dbl)
      n297 = Index Array(array=w872, index=w797) -> (element=w854:dbl)
      n298 = Index Array(array=w804, index=w796) -> (element=w822:dbl)
      n299 = Index Array(array=w761, index=w795) -> (element=w779:dbl)
      n300 = Index Array(array=w750, index=w716) -> (element=w732:dbl)
      n301 = Index Array(array=w592, index=w556) -> (element=w574:dbl)
      n302 = Index Array(array=w869, index=w797) -> (element=w851:dbl)
      n303 = Index Array(array=w598, index=w635) -> (element=w616:dbl)
      n304 = Index Array(array=w591, index=w556) -> (element=w573:dbl)
      n305 = Index Array(array=w587, index=w556) -> (element=w569:dbl)
      n306 = Index Array(array=w518, index=w555) -> (element=w536:dbl)
      n307 = Index Array(array=w759, index=w795) -> (element=w777:dbl)
      n308 = Index Array(array=w752, index=w716) -> (element=w734:dbl)
      n309 = Index Array(array=w871, index=w797) -> (element=w853:dbl)
      n310 = Index Array(array=w760, index=w795) -> (element=w778:dbl)
      n311 = Index Array(array=w764, index=w795) -> (element=w782:dbl)
      n312 = Index Array(array=w751, index=w716) -> (element=w733:dbl)
      n313 = Index Array(array=w747, index=w716) -> (element=w729:dbl)
      n314 = Index Array(array=w601, index=w635) -> (element=w619:dbl)
      n315 = Index Array(array=w589, index=w556) -> (element=w571:dbl)
      n316 = Index Array(array=w521, index=w555) -> (element=w539:dbl)
      n317 = Index Array(array=w870, index=w797) -> (element=w852:dbl)
      n318 = Index Array(array=w866, index=w797) -> (element=w848:dbl)
      n319 = Index Array(array=w588, index=w556) -> (element=w570:dbl)
      n320 = Index Array(array=w762, index=w795) -> (element=w780:dbl)
      n321 = Index Array(array=w749, index=w716) -> (element=w731:dbl)
      n322 = Index Array(array=w676, index=w715) -> (element=w677:dbl)
      n323 = Index Array(array=w675, index=w636) -> (element=w674:dbl)
      n324 = Index Array(array=w599, index=w635) -> (element=w617:dbl)
      n325 = Index Array(array=w519, index=w555) -> (element=w537:dbl)
      n326 = Index Array(array=w868, index=w797) -> (element=w850:dbl)
      n327 = Index Array(array=w763, index=w795) -> (element=w781:dbl)
      n328 = Index Array(array=w748, index=w716) -> (element=w730:dbl)
      n329 = Index Array(array=w600, index=w635) -> (element=w618:dbl)
      n330 = Index Array(array=w604, index=w635) -> (element=w622:dbl)
      n331 = Index Array(array=w520, index=w555) -> (element=w538:dbl)
      n332 = Index Array(array=w524, index=w555) -> (element=w542:dbl)
      n333 = Index Array(array=w867, index=w797) -> (element=w849:dbl)
      n334 = Index Array(array=w685, index=w715) -> (element=w703:dbl)
      n335 = Index Array(array=w666, index=w636) -> (element=w648:dbl)
      n336 = Index Array(array=w602, index=w635) -> (element=w620:dbl)
      n337 = Index Array(array=w522, index=w555) -> (element=w540:dbl)
      n338 = Index Array(array=w603, index=w635) -> (element=w621:dbl)
      n339 = Index Array(array=w523, index=w555) -> (element=w541:dbl)
      n340 = Index Array(array=w678, index=w715) -> (element=w696:dbl)
      n341 = Index Array(array=w673, index=w636) -> (element=w655:dbl)
      n342 = Index Array(array=w681, index=w715) -> (element=w699:dbl)
      n343 = Index Array(array=w670, index=w636) -> (element=w652:dbl)
      n344 = Index Array(array=w679, index=w715) -> (element=w697:dbl)
      n345 = Index Array(array=w672, index=w636) -> (element=w654:dbl)
      n346 = Index Array(array=w680, index=w715) -> (element=w698:dbl)
      n347 = Index Array(array=w684, index=w715) -> (element=w702:dbl)
      n348 = Index Array(array=w671, index=w636) -> (element=w653:dbl)
      n349 = Index Array(array=w667, index=w636) -> (element=w649:dbl)
      n350 = Index Array(array=w682, index=w715) -> (element=w700:dbl)
      n351 = Index Array(array=w669, index=w636) -> (element=w651:dbl)
      n352 = Index Array(array=w683, index=w715) -> (element=w701:dbl)
      n353 = Index Array(array=w668, index=w636) -> (element=w650:dbl)
      n354 = local read "PWM10"() -> (w815:dbl[])
      n355 = local read "PWM18"() -> (w807:dbl[])
      n356 = local read "PWM10"() -> (w577:dbl[])
      n357 = local read "PWM11"() -> (w814:dbl[])
      n358 = local read "PWM10"() -> (w774:dbl[])
      n359 = local read "PWM10"() -> (w737:dbl[])
      n360 = local read "PWM18"() -> (w585:dbl[])
      n361 = local read "PWM14"() -> (w811:dbl[])
      n362 = local read "PWM10"() -> (w856:dbl[])
      n363 = local read "PWM18"() -> (w766:dbl[])
      n364 = local read "PWM18"() -> (w745:dbl[])
      n365 = local read "PWM12"() -> (w813:dbl[])
      n366 = local read "PWM18"() -> (w864:dbl[])
      n367 = local read "PWM10"() -> (w614:dbl[])
      n368 = local read "PWM11"() -> (w578:dbl[])
      n369 = local read "PWM10"() -> (w534:dbl[])
      n370 = local read "PWM13"() -> (w812:dbl[])
      n371 = local read "PWM17"() -> (w808:dbl[])
      n372 = local read "PWM11"() -> (w773:dbl[])
      n373 = local read "PWM11"() -> (w738:dbl[])
      n374 = local read "PWM18"() -> (w606:dbl[])
      n375 = local read "PWM14"() -> (w581:dbl[])
      n376 = local read "PWM18"() -> (w526:dbl[])
      n377 = local read "PWM15"() -> (w810:dbl[])
      n378 = local read "PWM11"() -> (w857:dbl[])
      n379 = local read "PWM16"() -> (w809:dbl[])
      n380 = local read "PWM14"() -> (w770:dbl[])
      n381 = local read "PWM14"() -> (w741:dbl[])
      n382 = local read "PWM12"() -> (w579:dbl[])
      n383 = local read "PWM14"() -> (w860:dbl[])
      n384 = local read "PWM11"() -> (w613:dbl[])
      n385 = local read "PWM13"() -> (w580:dbl[])
      n386 = local read "PWM17"() -> (w584:dbl[])
      n387 = local read "PWM11"() -> (w533:dbl[])
      n388 = local read "PWM12"() -> (w772:dbl[])
      n389 = local read "PWM12"() -> (w739:dbl[])
      n390 = local read "PWM12"() -> (w858:dbl[])
      n391 = local read "PWM13"() -> (w771:dbl[])
      n392 = local read "PWM17"() -> (w767:dbl[])
      n393 = local read "PWM13"() -> (w740:dbl[])
      n394 = local read "PWM17"() -> (w744:dbl[])
      n395 = local read "PWM14"() -> (w610:dbl[])
      n396 = local read "PWM15"() -> (w582:dbl[])
      n397 = local read "PWM14"() -> (w530:dbl[])
      n398 = local read "PWM13"() -> (w859:dbl[])
      n399 = local read "PWM17"() -> (w863:dbl[])
      n400 = local read "PWM16"() -> (w583:dbl[])
      n401 = local read "PWM15"() -> (w769:dbl[])
      n402 = local read "PWM15"() -> (w742:dbl[])
      n403 = local read "PWM10"() -> (w694:dbl[])
      n404 = local read "PWM10"() -> (w657:dbl[])
      n405 = local read "PWM12"() -> (w612:dbl[])
      n406 = local read "PWM12"() -> (w532:dbl[])
      n407 = local read "PWM15"() -> (w861:dbl[])
      n408 = local read "PWM16"() -> (w768:dbl[])
      n409 = local read "PWM16"() -> (w743:dbl[])
      n410 = local read "PWM13"() -> (w611:dbl[])
      n411 = local read "PWM17"() -> (w607:dbl[])
      n412 = local read "PWM13"() -> (w531:dbl[])
      n413 = local read "PWM17"() -> (w527:dbl[])
      n414 = local read "PWM16"() -> (w862:dbl[])
      n415 = local read "PWM18"() -> (w686:dbl[])
      n416 = local read "PWM18"() -> (w665:dbl[])
      n417 = local read "PWM15"() -> (w609:dbl[])
      n418 = local read "PWM15"() -> (w529:dbl[])
      n419 = local read "PWM16"() -> (w608:dbl[])
      n420 = local read "PWM16"() -> (w528:dbl[])
      n421 = local read "PWM11"() -> (w693:dbl[])
      n422 = local read "PWM11"() -> (w658:dbl[])
      n423 = local read "PWM14"() -> (w690:dbl[])
      n424 = local read "PWM14"() -> (w661:dbl[])
      n425 = local read "PWM12"() -> (w692:dbl[])
      n426 = local read "PWM12"() -> (w659:dbl[])
      n427 = local read "PWM13"() -> (w691:dbl[])
      n428 = local read "PWM17"() -> (w687:dbl[])
      n429 = local read "PWM13"() -> (w660:dbl[])
      n430 = local read "PWM17"() -> (w664:dbl[])
      n431 = local read "PWM15"() -> (w689:dbl[])
      n432 = local read "PWM15"() -> (w662:dbl[])
      n433 = local read "PWM16"() -> (w688:dbl[])
      n434 = local read "PWM16"() -> (w663:dbl[])
      n435 = Index Array(array=w815, index=w796) -> (element=w825:dbl)
      n436 = Index Array(array=w807, index=w796) -> (element=w833:dbl)
      n437 = Index Array(array=w577, index=w556) -> (element=w567:dbl)
      n438 = Index Array(array=w814, index=w796) -> (element=w826:dbl)
      n439 = Index Array(array=w774, index=w795) -> (element=w784:dbl)
      n440 = Index Array(array=w737, index=w716) -> (element=w727:dbl)
      n441 = Index Array(array=w585, index=w556) -> (element=w559:dbl)
      n442 = Index Array(array=w811, index=w796) -> (element=w829:dbl)
      n443 = Index Array(array=w856, index=w797) -> (element=w846:dbl)
      n444 = Index Array(array=w766, index=w795) -> (element=w792:dbl)
      n445 = Index Array(array=w745, index=w716) -> (element=w719:dbl)
      n446 = Index Array(array=w813, index=w796) -> (element=w827:dbl)
      n447 = Index Array(array=w864, index=w797) -> (element=w838:dbl)
      n448 = Index Array(array=w614, index=w635) -> (element=w624:dbl)
      n449 = Index Array(array=w578, index=w556) -> (element=w566:dbl)
      n450 = Index Array(array=w534, index=w555) -> (element=w544:dbl)
      n451 = Index Array(array=w812, index=w796) -> (element=w828:dbl)
      n452 = Index Array(array=w808, index=w796) -> (element=w832:dbl)
      n453 = Index Array(array=w773, index=w795) -> (element=w785:dbl)
      n454 = Index Array(array=w738, index=w716) -> (element=w726:dbl)
      n455 = Index Array(array=w606, index=w635) -> (element=w632:dbl)
      n456 = Index Array(array=w581, index=w556) -> (element=w563:dbl)
      n457 = Index Array(array=w526, index=w555) -> (element=w552:dbl)
      n458 = Index Array(array=w810, index=w796) -> (element=w830:dbl)
      n459 = Index Array(array=w857, index=w797) -> (element=w845:dbl)
      n460 = Index Array(array=w809, index=w796) -> (element=w831:dbl)
      n461 = Index Array(array=w770, index=w795) -> (element=w788:dbl)
      n462 = Index Array(array=w741, index=w716) -> (element=w723:dbl)
      n463 = Index Array(array=w579, index=w556) -> (element=w565:dbl)
      n464 = Index Array(array=w860, index=w797) -> (element=w842:dbl)
      n465 = Index Array(array=w613, index=w635) -> (element=w625:dbl)
      n466 = Index Array(array=w580, index=w556) -> (element=w564:dbl)
      n467 = Index Array(array=w584, index=w556) -> (element=w560:dbl)
      n468 = Index Array(array=w533, index=w555) -> (element=w545:dbl)
      n469 = Index Array(array=w772, index=w795) -> (element=w786:dbl)
      n470 = Index Array(array=w739, index=w716) -> (element=w725:dbl)
      n471 = Index Array(array=w858, index=w797) -> (element=w844:dbl)
      n472 = Index Array(array=w771, index=w795) -> (element=w787:dbl)
      n473 = Index Array(array=w767, index=w795) -> (element=w791:dbl)
      n474 = Index Array(array=w740, index=w716) -> (element=w724:dbl)
      n475 = Index Array(array=w744, index=w716) -> (element=w720:dbl)
      n476 = Index Array(array=w610, index=w635) -> (element=w628:dbl)
      n477 = Index Array(array=w582, index=w556) -> (element=w562:dbl)
      n478 = Index Array(array=w530, index=w555) -> (element=w548:dbl)
      n479 = Index Array(array=w859, index=w797) -> (element=w843:dbl)
      n480 = Index Array(array=w863, index=w797) -> (element=w839:dbl)
      n481 = Index Array(array=w583, index=w556) -> (element=w561:dbl)
      n482 = Index Array(array=w769, index=w795) -> (element=w789:dbl)
      n483 = Index Array(array=w742, index=w716) -> (element=w722:dbl)
      n484 = Index Array(array=w694, index=w715) -> (element=w704:dbl)
      n485 = Index Array(array=w657, index=w636) -> (element=w647:dbl)
      n486 = Index Array(array=w612, index=w635) -> (element=w626:dbl)
      n487 = Index Array(array=w532, index=w555) -> (element=w546:dbl)
      n488 = Index Array(array=w861, index=w797) -> (element=w841:dbl)
      n489 = Index Array(array=w768, index=w795) -> (element=w790:dbl)
      n490 = Index Array(array=w743, index=w716) -> (element=w721:dbl)
      n491 = Index Array(array=w611, index=w635) -> (element=w627:dbl)
      n492 = Index Array(array=w607, index=w635) -> (element=w631:dbl)
      n493 = Index Array(array=w531, index=w555) -> (element=w547:dbl)
      n494 = Index Array(array=w527, index=w555) -> (element=w551:dbl)
      n495 = Index Array(array=w862, index=w797) -> (element=w840:dbl)
      n496 = Index Array(array=w686, index=w715) -> (element=w712:dbl)
      n497 = Index Array(array=w665, index=w636) -> (element=w639:dbl)
      n498 = Index Array(array=w609, index=w635) -> (element=w629:dbl)
      n499 = Index Array(array=w529, index=w555) -> (element=w549:dbl)
      n500 = Index Array(array=w608, index=w635) -> (element=w630:dbl)
      n501 = Index Array(array=w528, index=w555) -> (element=w550:dbl)
      n502 = Index Array(array=w693, index=w715) -> (element=w705:dbl)
      n503 = Index Array(array=w658, index=w636) -> (element=w646:dbl)
      n504 = Index Array(array=w690, index=w715) -> (element=w708:dbl)
      n505 = Index Array(array=w661, index=w636) -> (element=w643:dbl)
      n506 = Index Array(array=w692, index=w715) -> (element=w706:dbl)
      n507 = Index Array(array=w659, index=w636) -> (element=w645:dbl)
      n508 = Index Array(array=w691, index=w715) -> (element=w707:dbl)
      n509 = Index Array(array=w687, index=w715) -> (element=w711:dbl)
      n510 = Index Array(array=w660, index=w636) -> (element=w644:dbl)
      n511 = Index Array(array=w664, index=w636) -> (element=w640:dbl)
      n512 = Index Array(array=w689, index=w715) -> (element=w709:dbl)
      n513 = Index Array(array=w662, index=w636) -> (element=w642:dbl)
      n514 = Index Array(array=w688, index=w715) -> (element=w710:dbl)
      n515 = Index Array(array=w663, index=w636) -> (element=w641:dbl)
      n516 = local read "PWM19"() -> (w816:dbl[])
      n517 = local read "PWM19"() -> (w576:dbl[])
      n518 = local read "PWM19"() -> (w775:dbl[])
      n519 = local read "PWM19"() -> (w736:dbl[])
      n520 = local read "PWM19"() -> (w855:dbl[])
      n521 = local read "PWM19"() -> (w615:dbl[])
      n522 = local read "PWM19"() -> (w535:dbl[])
      n523 = local read "PWM19"() -> (w695:dbl[])
      n524 = local read "PWM19"() -> (w656:dbl[])
      n525 = Index Array(array=w816, index=w796) -> (element=w834:dbl)
      n526 = Index Array(array=w576, index=w556) -> (element=w558:dbl)
      n527 = Index Array(array=w775, index=w795) -> (element=w793:dbl)
      n528 = Index Array(array=w736, index=w716) -> (element=w718:dbl)
      n529 = Index Array(array=w855, index=w797) -> (element=w837:dbl)
      n530 = Index Array(array=w615, index=w635) -> (element=w633:dbl)
      n531 = Index Array(array=w535, index=w555) -> (element=w553:dbl)
      n532 = Index Array(array=w695, index=w715) -> (element=w713:dbl)
      n533 = Index Array(array=w656, index=w636) -> (element=w638:dbl)
      n534 = Build Array(w798, w817, w818, w819, w820, w821, w822, w823, w824, w825, w826, w827, w828, w829, w830, w831, w832, w833, w834) -> (→"SENSOR1":dbl[])
      n535 = Build Array(w594, w575, w574, w573, w572, w571, w570, w569, w568, w567, w566, w565, w564, w563, w562, w561, w560, w559, w558) -> (→"SENSOR 8":dbl[])
      n536 = Build Array(w757, w776, w777, w778, w779, w780, w781, w782, w783, w784, w785, w786, w787, w788, w789, w790, w791, w792, w793) -> (→"SENSOR 3":dbl[])
      n537 = Build Array(w754, w735, w734, w733, w732, w731, w730, w729, w728, w727, w726, w725, w724, w723, w722, w721, w720, w719, w718) -> (→"SENSOR 4":dbl[])
      n538 = Build Array(w873, w854, w853, w852, w851, w850, w849, w848, w847, w846, w845, w844, w843, w842, w841, w840, w839, w838, w837) -> (→"SENSOR 2":dbl[])
      n539 = Build Array(w597, w616, w617, w618, w619, w620, w621, w622, w623, w624, w625, w626, w627, w628, w629, w630, w631, w632, w633) -> (→"SENSOR 7":dbl[])
      n540 = Build Array(w517, w536, w537, w538, w539, w540, w541, w542, w543, w544, w545, w546, w547, w548, w549, w550, w551, w552, w553) -> (→"SENSOR 9":dbl[])
      n541 = Build Array(w677, w696, w697, w698, w699, w700, w701, w702, w703, w704, w705, w706, w707, w708, w709, w710, w711, w712, w713) -> (→"SENSOR 5":dbl[])
      n542 = Build Array(w674, w655, w654, w653, w652, w651, w650, w649, w648, w647, w646, w645, w644, w643, w642, w641, w640, w639, w638) -> (→"SENSOR 6":dbl[])
    }
  }
